vi "Thingspeak-Amazon.vi"() -> ()   [LabVIEW 2017]
uses:
  <vilib>/Instr/_visa.llb/VISA Configure Serial Port (Instr).vi
  <vilib>/httpClient/LabVIEWHTTPClient.lvlib
panel:
  out "Thermometer":dbl(slide) scale=0.0..100.0
  out "Tank":dbl(slide) scale=0.0..100.0
  out "Temperatura":dbl
  out "Humedad":dbl
  in  "Puerto COM":refnum<visa-resource-name>
  out "Valor Recibido":string
  in  "API Key Thingspeak":string
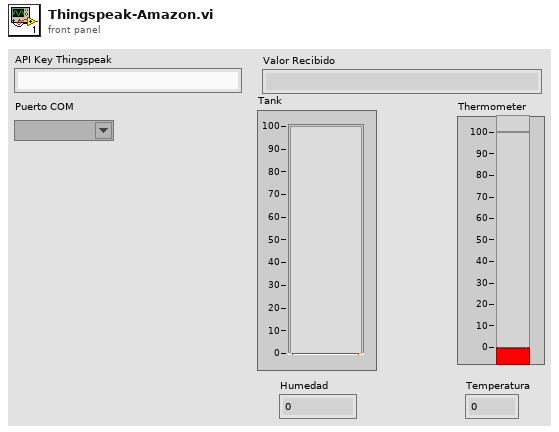
[diagram p1: front panel]
types:
  T1 = typedef "LabVIEWHTTPClient.lvlib/ClientHandle.ctl" = refnum<k1>
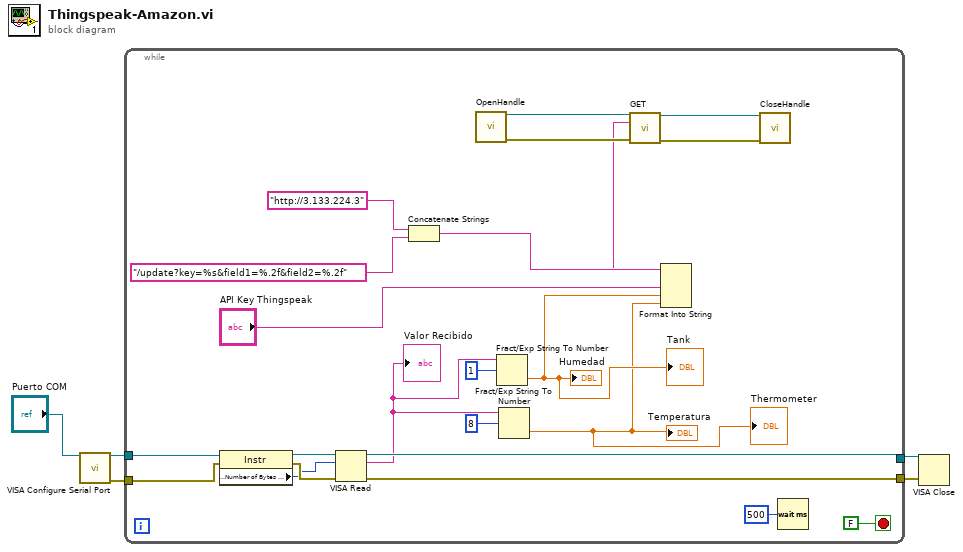
[diagram p0: block diagram]
diagram:
  n1 = call-poly "VISA Configure Serial Port"("VISA resource name"="Puerto COM") -> ("VISA resource name out"=w5:refnum<visa-resource-name>, "error out"=w4:errorcluster)  [unwired: 13 in]
  n2 = while {
    tunnel: w5 -> [w17]
    tunnel: w4 -> [w16]
    tunnel: [w12] -> w3
    tunnel: [w11] -> w2
    stop <- FALSE stop-if-true
    n3 = property class="Instr"(reference=w17, error in=w16) -> (reference out=w15:refnum<visa-resource-name>, error out=w14:errorcluster, "Serial Settings:Number of Bytes at Serial Port"=w13:u32)
    n4 = VISA Read(VISA resource name=w15, byte count=w13, error in (no error)=w14) -> (VISA resource name out=w12:refnum<visa-resource-name>, read buffer=w10:string, error out=w11:errorcluster)  [unwired: 1 out]
    "Valor Recibido" <- w10
    n5 = Concatenate Strings "Concatenate Strings"("http://3.133.224.3" ("string"), "/update?key=%s&field1=%.2f&field2=%.2f" ("string")) -> (w24:string)
    n6 = call <vilib>:"OpenHandle.vi"() -> ("client handle out"=w28:T1, "error out"=w25:errorcluster)  [unwired: 14 in]
    n7 = Fract/Exp String To Number(string=w10, offset=1) -> (number=w7:dbl)  [unwired: 2 in, 1 out]
    "Humedad" <- w7
    "Tank" <- w7
    n8 = Fract/Exp String To Number(string=w10, offset=8) -> (number=w6:dbl)  [unwired: 2 in, 1 out]
    "Temperatura" <- w6
    "Thermometer" <- w6
    n9 = Format Into String "Format Into String"(format string=w24, "API Key Thingspeak", w7, w6) -> (resulting string=w21:string)  [unwired: 2 in, 1 out]
    n10 = call <vilib>:"GET.vi"("client handle"=w28, "url"=w21, "error in (no error)"=w25) -> ("client handle out"=w27:T1, "error out"=w26:errorcluster)  [unwired: 9 in, 2 out]
    n11 = call <vilib>:"CloseHandle.vi"("client handle"=w27, "error in (no error)"=w26) -> ()  [unwired: 13 in, 1 out]
    n12 = Wait (ms)(milliseconds to wait=u32 500) -> ()  [unwired: 1 out]
  }
  n13 = VISA Close(VISA resource name=w3, error in (no error)=w2) -> ()  [unwired: 1 out]
